vi "main.vi"() -> ()   [LabVIEW 2021]
uses:
  Peasant/PeasantCluster.ctl
  Peasant/Peasant.lvclass
  Peasant/Peasant.lvclass/Peasant.ctl
  Peasant/Read Peasant Attributes.vi
  Peasant/Write Peasant Attributes.vi
panel:
  out "Tank":dbl(slide) scale=0.0..20.0
  out "Attack 1":i32(knob) scale=0.0..13.0
  out "Attack 2":dbl(knob) scale=0.0..10.0
  out "error out":errorcluster
  out "Cube 2":i32
  out "Cube 1":i32
  in  "Attack 2":bool
  in  "Attack 1":bool
  in  "Stop":bool
  out "Peasant 2":T1
  out "Peasant 1":T1
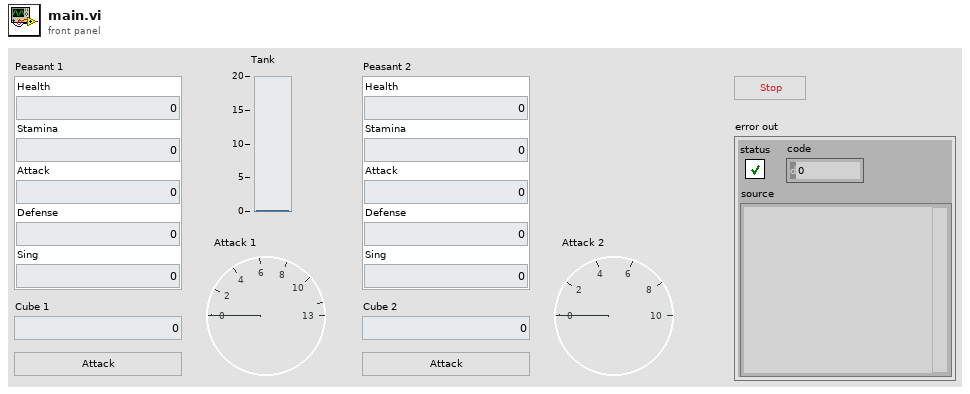
[diagram p1: front panel]
types:
  T1 = typedef "PeasantCluster.ctl" = cluster{"Health":i32, "Stamina":i32, "Attack":i32, "Defense":i32, "Sing":i32}
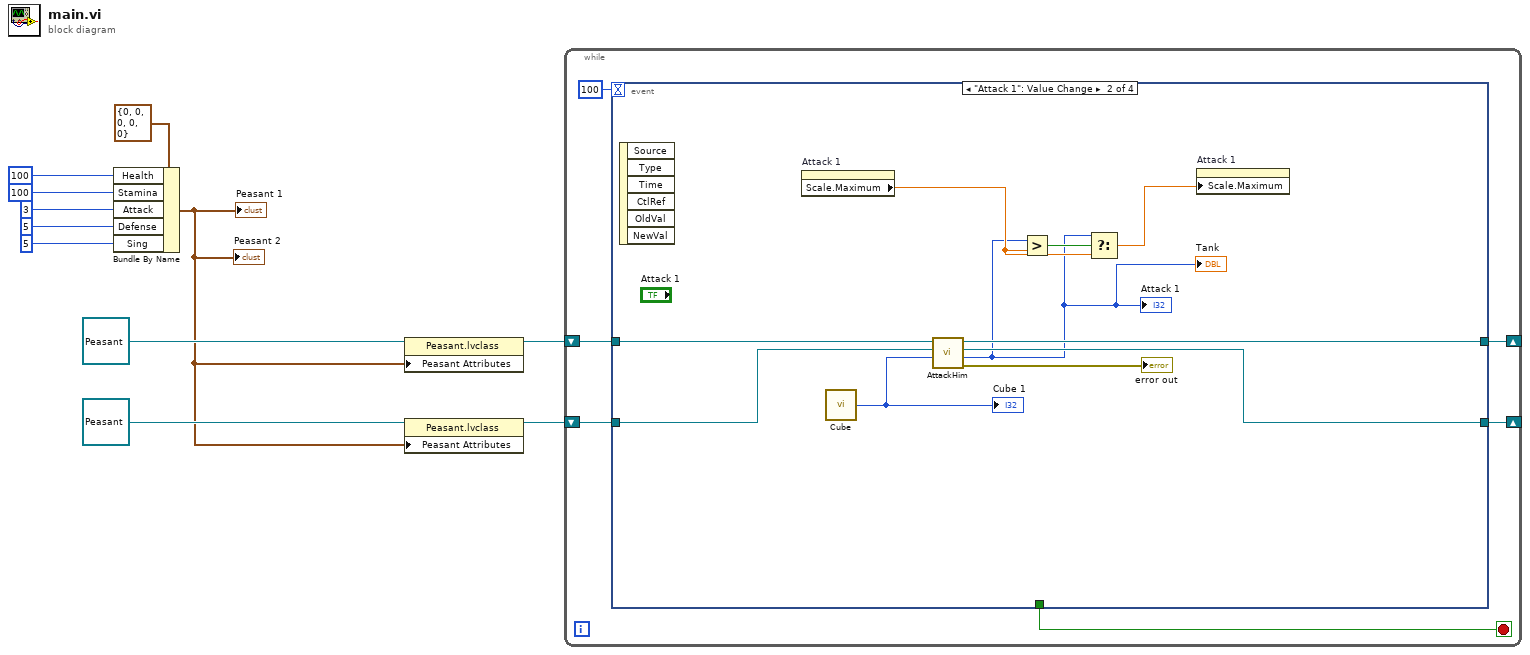
[diagram p0: block diagram]
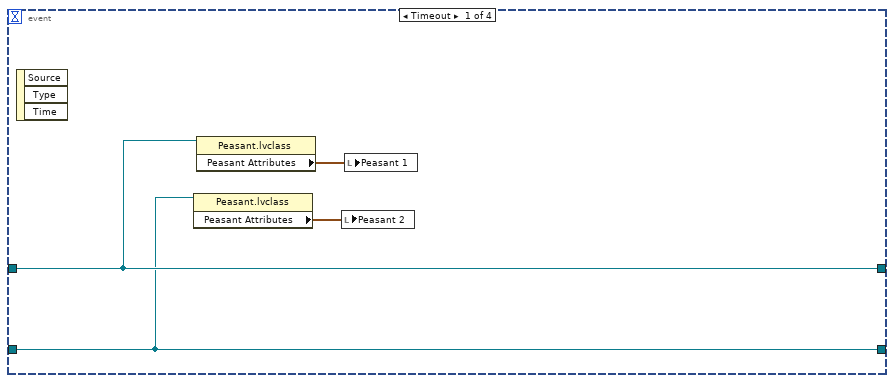
[diagram p2: hidden frame]
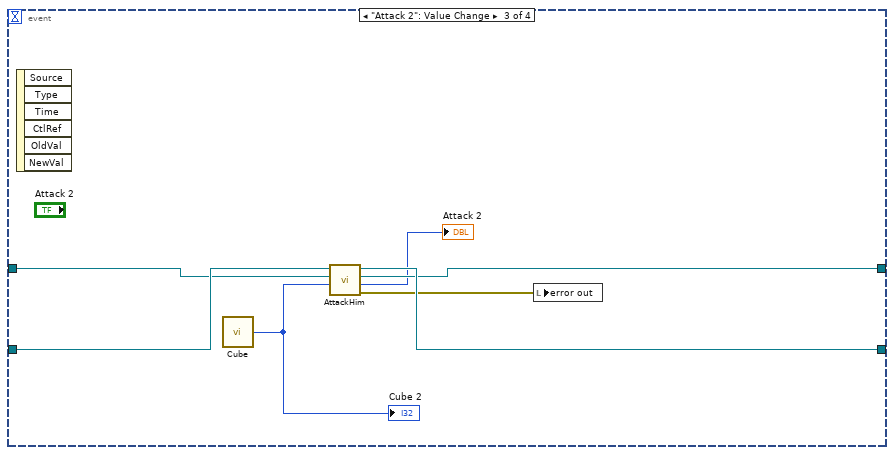
[diagram p3: hidden frame]
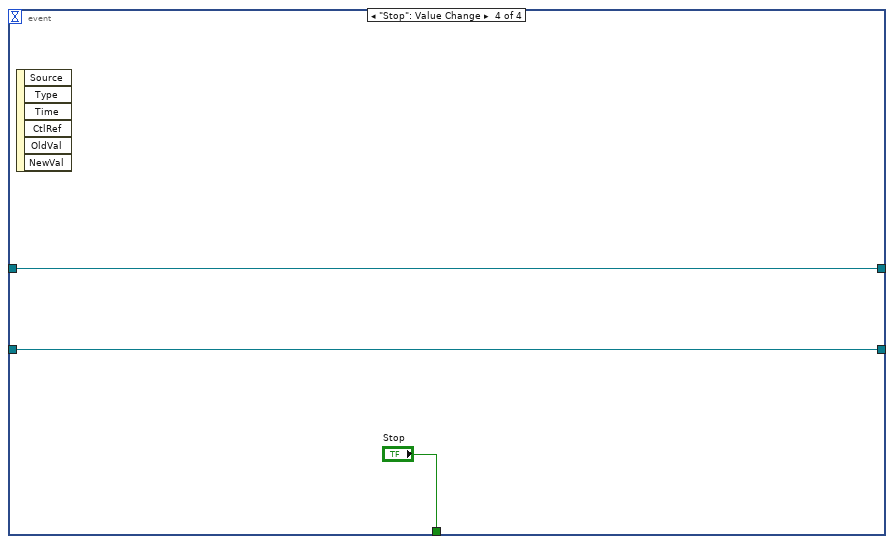
[diagram p4: hidden frame]
diagram:
  n1 = Bundle By Name(cluster=T1 {"Health"=0, "Stamina"=0, "Attack"=0, "Defense"=0, "Sing"=0} ("Peasant 1"), "Health"=100, "Stamina"=100, "Attack"=3, "Defense"=5, "Sing"=5) -> (w4:T1)
  "Peasant 1" <- w4
  "Peasant 2" <- w4
  n2 = property class="Peasant.lvclass"(reference=refnum<class "Peasant.lvclass"> refnum ("Peasant.lvclass"), "Peasant Attributes"=w4) -> (reference out=w3:refnum<class "Peasant.lvclass">)  [unwired: 1 in, 1 out]
  n3 = property class="Peasant.lvclass"(reference=refnum<class "Peasant.lvclass"> refnum ("Peasant.lvclass"), "Peasant Attributes"=w4) -> (reference out=w2:refnum<class "Peasant.lvclass">)  [unwired: 1 in, 1 out]
  n4 = while {
    shift-right: [w13] -> _
    shift-left: w3 -> [w14]
    shift-right: [w15] -> _
    shift-left: w2 -> [w16]
    stop <- w17 stop-if-true
    n5 = event shown="[1] \"Attack 1\": Value Change" {
      selector: _ -> [_ _ _ _]
      dyn-events: _ -> [_ _ _ _]
      timeout: 100 -> [_ _ _ _]
      tunnel: [_ _ _ "Stop"] -> w17
      tunnel: w16 -> [w19 w30 w38 w40]
      tunnel: [w19 w28 w36 w40] -> w15
      tunnel: w14 -> [w21 w31 w37 w39]
      tunnel: [w21 w29 w35 w39] -> w13
      event Timeout {
        n6 = event-data() -> ()  [unwired: 1 in, 3 out]
        n7 = property class="Peasant.lvclass"(reference=w19) -> ("Peasant Attributes"=w18:T1)  [unwired: 1 in, 2 out]
        n8 = property class="Peasant.lvclass"(reference=w21) -> ("Peasant Attributes"=w20:T1)  [unwired: 1 in, 2 out]
        n9 = local write "Peasant 2"(w18) -> ()
        n10 = local write "Peasant 1"(w20) -> ()
      }
      event "Attack 1": Value Change {
        n11 = event-data() -> ()  [unwired: 1 in, 6 out]
        n12 = property on="Attack 1" class="Knob (strict)"() -> ("Scale.Maximum"=w24:dbl)  [unwired: 2 in, 2 out]
        n13 = call "Cube.vi"() -> ("Number"=w27:u64)
        "Cube 1" <- w27
        n14 = call-dynamic "AttackHim.vi"("Cube"=w27, "Rival"=w30, "Peasant in"=w31) -> ("error out"=→"error out":errorcluster, "CurrentAttack"=w22:i32, "Rival out"=w28:refnum<class "Peasant.lvclass">, "Peasant out"=w29:refnum<class "Peasant.lvclass">)  [unwired: 5 in]
        "Attack 1" <- w22
        "Tank" <- w22
        n15 = Greater?(x=w22, y=w24) -> (0:w25:bool)
        n16 = Select(t=w22, s=w25, f=w24) -> (s? t:f=w23:dbl)
        n17 = property on="Attack 1" class="Knob (strict)"("Scale.Maximum"=w23) -> ()  [unwired: 2 in, 2 out]
      }
      event "Attack 2": Value Change {
        n18 = event-data() -> ()  [unwired: 1 in, 6 out]
        n19 = call "Cube.vi"() -> ("Number"=w34:u64)
        "Cube 2" <- w34
        n20 = call-dynamic "AttackHim.vi"("Cube"=w34, "Rival"=w37, "Peasant in"=w38) -> ("error out"=w33:errorcluster, "CurrentAttack"=→"Attack 2":i32, "Rival out"=w35:refnum<class "Peasant.lvclass">, "Peasant out"=w36:refnum<class "Peasant.lvclass">)  [unwired: 5 in]
        n21 = local write "error out"(w33) -> ()
      }
      event "Stop": Value Change {
        n22 = event-data() -> ()  [unwired: 1 in, 6 out]
      }
    }
  }
